vi "Update UEGO Cards.vi"(8 "error in (no error)":errorcluster, 10 "Bitfile Info":T1, 11 "Device Ref in":T2 format="%.0x") -> (0 "error out":errorcluster)   [LabVIEW 2014, in "SLSC configuration System Explorer.lvlib"]
uses:
  SLSC configuration System Explorer.lvlib
  <vilib>/NI Veristand/Custom Device API/Custom Device Item Ref.ctl
  Type Defs/SLSC Bitfile Info.ctl
  Shared/Constants.vi
  <vilib>/NI Veristand/Custom Device API/Get Item Property (String).vi
  <vilib>/NI Veristand/Custom Device API/Custom Device API.lvlib
  Shared/SLSC configuration Shared.lvlib
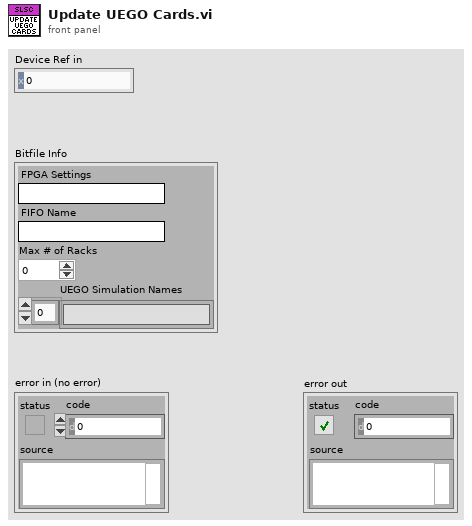
[diagram p1: front panel]
types:
  T1 = typedef "SLSC configuration System Explorer.lvlib/SLSC Bitfile Info.ctl" = cluster{"FPGA Settings":string, "FIFO Name":string, "Max # of Racks":u8, "UEGO Simulation Names":string[]}
  T2 = typedef "Custom Device API.lvlib/Custom Device Item Ref.ctl" = u64
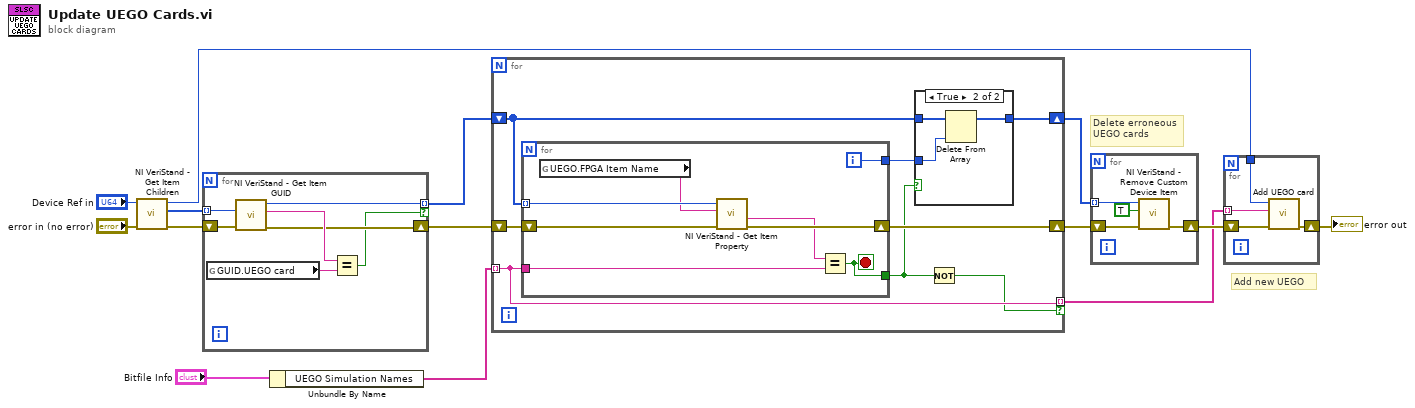
[diagram p0: block diagram]
diagram:
  # "Add new UEGO"
  # "Delete erroneous\nUEGO cards"
  n1 = call <vilib>:"NI VeriStand - Get Item Children.vi"("error in (no error)"="error in (no error)", "Item Ref in"="Device Ref in") -> ("error out"=w14:errorcluster, "Child Refs"=w10:T2[], "Item Ref out"=w1:T2)  [unwired: 6 in, 1 out]
  n2 = for {
    tunnel: w10 -> [w20] mode=indexing
    shift-right: [w17] -> w7
    shift-left: w14 -> [w19]
    tunnel: [w16] -> w9 mode=indexing if=w15
    n3 = global read "Constants.vi" "GUID.UEGO card"() -> (w21:string)
    n4 = call <vilib>:"NI VeriStand - Get Item GUID.vi"("error in (no error)"=w19, "Item Ref in"=w20) -> ("error out"=w17:errorcluster, "GUID"=w18:string, "Item Ref out"=w16:T2)  [unwired: 7 in]
    n5 = Equal?(x=w18, y=w21) -> (x = y?=w15:bool)
  }
  n6 = Unbundle By Name("Bitfile Info") -> ("UEGO Simulation Names"=w8:string[])
  n7 = for {
    shift-right: [w23] -> w5
    shift-left: w9 -> [w25]
    tunnel: w8 -> [w27] mode=indexing
    shift-right: [w28] -> w6
    shift-left: w7 -> [w29]
    tunnel: [w27] -> w2 mode=indexing if=w26
    n8 = for {
      tunnel: w27 -> [w36]
      tunnel: w25 -> [w40] mode=indexing
      shift-right: [w39] -> w28
      shift-left: w29 -> [w41]
      tunnel: [w35] -> w22
      tunnel: [w34] -> w24
      i -> [w34]
      stop <- w35 stop-if-true
      n9 = global read "Constants.vi" "UEGO.FPGA Item Name"() -> (w38:string)
      n10 = call-poly <vilib>:"NI VeriStand - Get Item Property.vi"("error in (no error)"=w41, "Property Name"=w38, "Item Ref in"=w40) -> ("error out"=w39:errorcluster, "Value"=w37:string)  [unwired: 5 in, 2 out]
      n11 = Equal?(x=w37, y=w36) -> (x = y?=w35:bool)
    }
    n12 = case shown="True" w22 {
      tunnel: w25 -> [w30 w33]
      tunnel: w24 -> [_ w32]
      tunnel: [w30 w31] -> w23
      frame False {
      }
      frame True {
        n13 = Delete From Array(array=w33, index=w32) -> (array with subset deleted=w31:T2[])  [unwired: 1 in, 1 out]
      }
    }
    n14 = Not(x=w22) -> (.not. x?=w26:bool)
  }
  n15 = for {
    tunnel: w5 -> [w43] mode=indexing
    shift-right: [w42] -> w4
    shift-left: w6 -> [w44]
    n16 = call <vilib>:"NI VeriStand - Remove Custom Device Item.vi"("error in (no error)"=w44, "Force Delete (F)"=TRUE, "Item Ref in"=w43) -> ("error out"=w42:errorcluster)  [unwired: 7 in, 1 out]
  }
  n17 = for {
    shift-right: [w48] -> w3
    shift-left: w4 -> [w49]
    tunnel: w2 -> [w47] mode=indexing
    tunnel: w1 -> [w46]
    n18 = call "Add UEGO card.vi"("error in (no error)"=w49, "FPGA Item Name"=w47, "Node Ptr"=w46) -> ("error out"=w48:errorcluster)  [unwired: 8 in]
  }
  "error out" <- w3
